vi "Get Points (1D).vi"(0 "eye scan point iterator":refnum<class "niHighSpeedSerial Rectangular Eye Scan Point Iterator v1 Host.lvclass">, 11 "error in":errorcluster) -> (4 "eye scan point iterator out":refnum<class "niHighSpeedSerial Rectangular Eye Scan Point Iterator v1 Host.lvclass">, 6 "array of points":T1[](array[typedef]), 15 "error out":errorcluster)   [LabVIEW 2014, in "niHighSpeedSerial Rectangular Eye Scan Point Iterator v1 Host.lvclass"]
doc: "Retrieves the points which have already been measured in a 1D array.\n\n<B>Input Parameters</B>\n\n<B>eye scan point iterator</B> is the incoming wire for the Eye Scan Point Iterator class object\n\n<B>error in</B> describes error conditions that occur before this node runs. This input provides standard 'error in' functionality.\n\n<B>Output Parameters</B>\n\n<B>eye scan point iterator out</B> is the outgoing wire for the Eye Scan Point Iterator class object\n\n<B>array of points</B> contains information related to each point, including its offsets, bit error rate, sample count, and error rate.\n\n<B>array of points.point offsets</B> contains the horizontal and vertical offsets for a point.\n\n<B>array of points.point offsets.horizontal offset</B> is the horizontal (unit interval) offset of a point.\n\n<B>array of points.point offsets.vertical offset</B> is the vertical (uncalibrated voltage) offset of a point.\n\n<B>array of points.sample count</B> is the number of samples measured.\n\n<B>array of points.error count</B> is the number of errors detected while measuring the point.\n\n<B>array of points.bit error rate</B> is the calculated statistical bit error rate based on the number of error counts and sample counts received.\n\n<B>error out</B> contains error information. This output provides standard 'error out' functionality."
uses:
  <instrlib>/niHighSpeedSerial/Eye Scan/v1/Host/Impl/Rect Iter/niHighSpeedSerial Rectangular Eye Scan Point Iterator v1 Host.lvclass
  <instrlib>/niHighSpeedSerial/Eye Scan/v1/Host/Common/Public/Point.ctl
  <instrlib>/niHighSpeedSerial/Eye Scan/v1/Host/Common/Public/Point Offsets.ctl
  <instrlib>/niHighSpeedSerial/Eye Scan/v1/Host/Impl/Rect Iter/niHighSpeedSerial Rectangular Eye Scan Point Iterator v1 Host.lvclass/niHighSpeedSerial Rectangular Eye Scan Point Iterator v1 Host.ctl
  <instrlib>/niHighSpeedSerial/Eye Scan/v1/Host/Common/niHighSpeedSerial Eye Scan Common v1 Host.lvlib
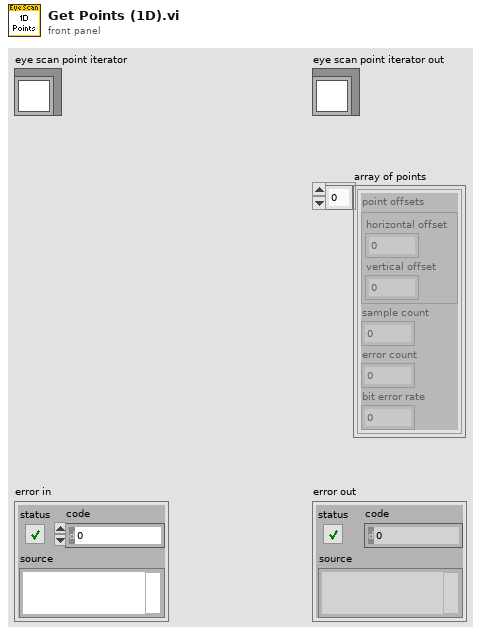
[diagram p1: front panel]
types:
  T1 = typedef "niHighSpeedSerial Eye Scan Common v1 Host.lvlib/Point.ctl" = cluster{"point offsets":T2, "sample count":u64, "error count":u64, "bit error rate":dbl}
  T2 = typedef "niHighSpeedSerial Eye Scan Common v1 Host.lvlib/Point Offsets.ctl" = cluster{"horizontal offset":i16, "vertical offset":i8}
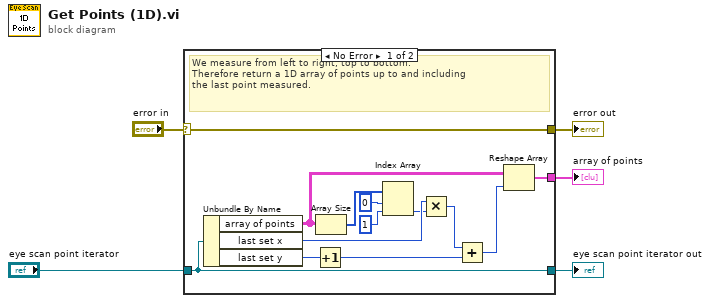
[diagram p0: block diagram]
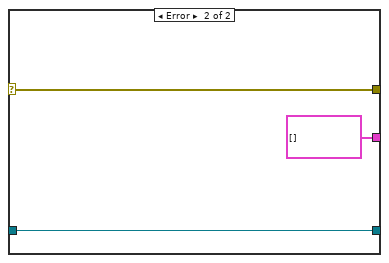
[diagram p2: hidden frame]
diagram:
  n1 = case shown="No Error" "error in" {
    selector: "error in" -> [w18 w21]
    tunnel: [w18 w21] -> w4
    tunnel: [w16 w20] -> w2
    tunnel: "eye scan point iterator" -> [w16 w20]
    tunnel: [w17 T1[] [] ("Array of Points")] -> w1
    frame No Error {
      # "We measure from left to right, top to bottom.\nTherefore return a 1D array of points up to and including\nthe last point measured."
      n2 = Unbundle By Name(w16) -> ("array of points"=w15:T1[][], "last set x"=w7:i32, "last set y"=w8:i32)
      n3 = Increment(x=w8) -> (x+1=w10:i32)
      n4 = Array Size(array=w15) -> (size(s)=w14:i32[])
      n5 = Index Array(array=w14, index #1=0 ("index"), index #2=1 ("index")) -> (element #2=w6:i32)  [unwired: 1 out]
      n6 = Multiply(x=w7, y=w6) -> (x*y=w11:i32)
      n7 = Add(x=w11, y=w10) -> (x+y=w9:i32)
      n8 = Reshape Array(w15, w9) -> (w17:T1[])
    }
    frame Error {
    }
  }
  "eye scan point iterator out" <- w2
  "error out" <- w4
  "array of points" <- w1
